vi "Test Syslog.vi"   [LabVIEW 2021]
uses:
  Source/abs_EventLog/Support/Facility Code.ctl
  Source/abs_EventLog/Support/Severity Code.ctl
  Source/Event_Syslog/Event_Syslog.lvclass
  C:/Users/Tim/Documents/GitHub/Event_log/Source/abs_EventLog/abs_EventLog.lvclass
  Source/abs_EventLog/abs_EventLog.lvclass/abs_EventLog.ctl
  Source/abs_EventLog/Properties/Write Facility Code.vi
  Source/abs_EventLog/Properties/Write Message Tag.vi
  Source/abs_EventLog/Properties/Write Severity Code.vi
  Source/abs_EventLog/abs_EventLog.lvclass
types:
  T1 = typedef "abs_EventLog.lvclass/Severity Code.ctl" = enum16{"emergency", "alert", "critical", "error", "warning", "notice", "info", "debug"}
  T2 = typedef "abs_EventLog.lvclass/Facility Code.ctl" = enum16{"kernel", "user", "mail", "system daemons", "security/authorization", "syslogd", "line printer", "network news", "uucp", "clock daemon", "security/authorization (alternate)", "FTP daemon", "NTP subsystem", "log audit", "log alert", "clock daemon (alternate)", "local use 0", "local use 1", "local use 2", "local use 3", "local use 4", "local use 5", "local use 6", "local use 7"}
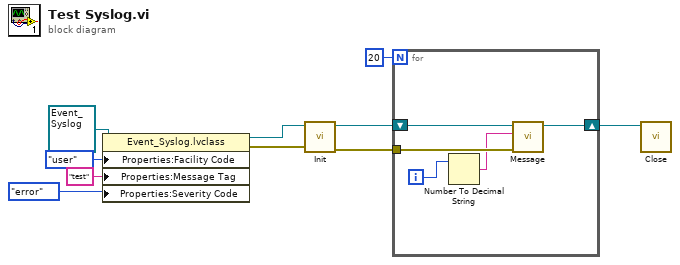
[diagram p0: block diagram]
diagram:
  n1 = property class="Event_Syslog.lvclass"(reference=refnum<class "Event_Syslog.lvclass"> refnum, "Properties:Facility Code"=Facility_Code."user" ("Facility Code"), "Properties:Message Tag"="test" ("Message Tag"), "Properties:Severity Code"=Severity_Code."error" ("Severity Code")) -> (reference out=w9:refnum<class "Event_Syslog.lvclass">, error out=w10:errorcluster)  [unwired: 1 in]
  n2 = call-dynamic "Init.vi"("error in (no error)"=w10, "Event_Syslog in"=w9) -> ("error out"=w5:errorcluster, "Event_Syslog out"=w4:refnum<class "Event_Syslog.lvclass">)  [unwired: 8 in]
  n3 = for {
    N: 20 -> [_]
    tunnel: w5 -> [w15]
    shift-right: [w13] -> w3
    shift-left: w4 -> [w14]
    i -> [w12]
    n4 = Number To Decimal String(number=w12) -> (decimal integer string=w11:string)  [unwired: 1 in]
    n5 = call-dynamic "Message.vi"("error in (no error)"=w15, "Message"=w11, "Syslog_Event in"=w14) -> ("Syslog_Event out"=w13:refnum<class "Event_Syslog.lvclass">)  [unwired: 7 in, 1 out]
  }
  n6 = call-dynamic "Close.vi"("Event_Syslog in"=w3) -> ()  [unwired: 9 in, 2 out]
